vi "GOMDBTS2048 get CRI Coordinates.vi"(8 "error in (no error)":errorcluster, 11 "handle":i32) -> (0 "error out":errorcluster, 2 "return type":i32, 3 "Cluster":cluster{"TLS":dbl[][], "RLS":dbl[][]})   [LabVIEW 2015, in "GOMDBTS2048.lvlib"]
uses:
  GOMDBTS2048.lvlib
  runtime/GOMDBTS2048.dll
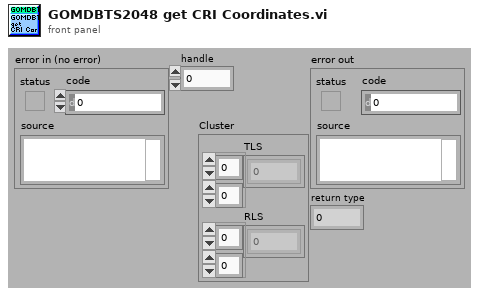
[diagram p1: front panel]
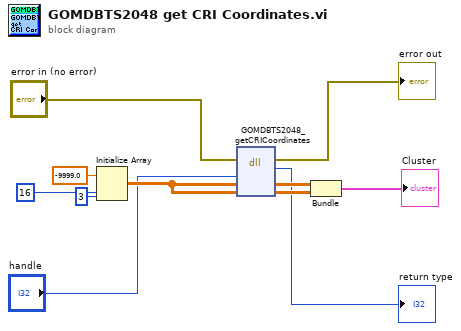
[diagram p0: block diagram]
diagram:
  n1 = Initialize Array(-9999.0 ("element"), 16 ("dimension size"), 3 ("dimension size")) -> (w8:dbl[][])
  n2 = dll-call lib="C:/Users/rkoch/Documents/GO_Library/runtime/GOMDBTS2048.dll" fn="GOMDBTS2048_getCRICoordinates"(error in="error in (no error)", "handle"="handle", "TLS"=w8, "RLS"=w8) -> (error out=→"error out":errorcluster, "return type"=→"return type":i32, "TLS"=w9:dbl[][], "RLS"=w10:dbl[][])  [unwired: 3 in, 1 out]
  n3 = Bundle("TLS"=w9, "RLS"=w10) -> (→"Cluster":cluster{"TLS":dbl[][], "RLS":dbl[][]})  [unwired: 1 in]
